vi "GeneralDataRequest.vi"(6 "Enable":bool, 8 "error in (no error)":errorcluster, 10 "Cluster":T2, 11 "VISA Refnum in":refnum<visa-resource-name>) -> (0 "error out":errorcluster, 3 "Sensor data":T1)   [LabVIEW 2020]
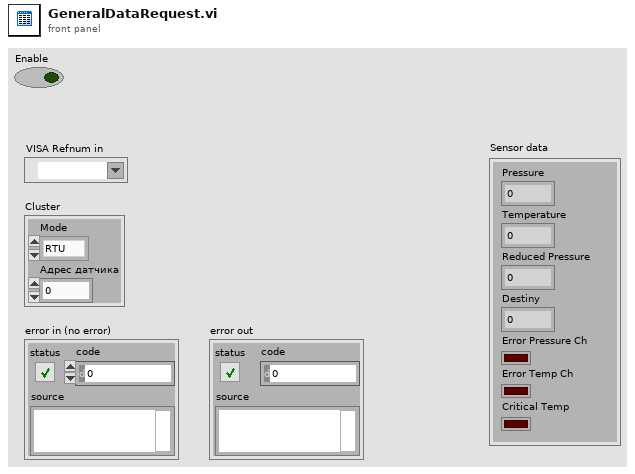
[diagram p1: front panel]
types:
  T1 = cluster{"Pressure":sgl, "Temperature":sgl, "Reduced Pressure":sgl, "Destiny":sgl, "Error Pressure Ch":bool, "Error Temp Ch":bool, "Critical Temp":bool}
  T2 = cluster{"Mode":enum16{"RTU", "ASCII"}, "Адрес датчика":u16}
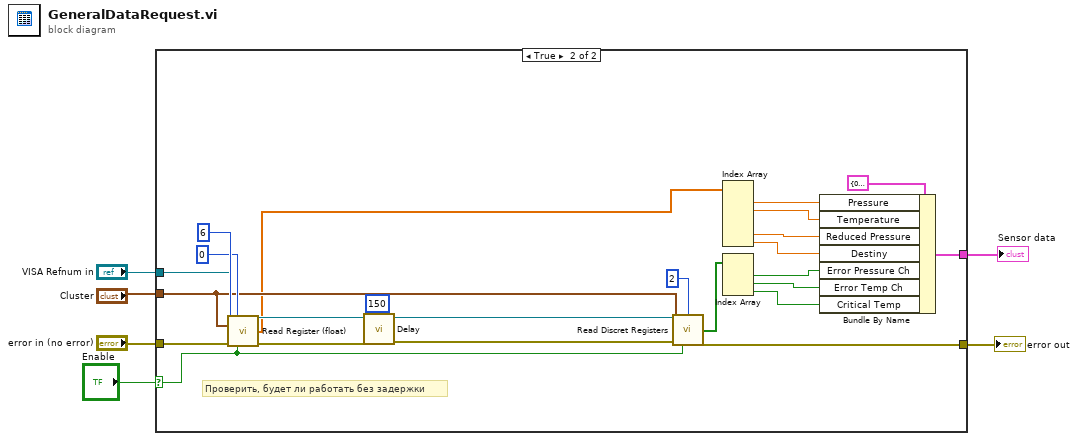
[diagram p0: block diagram]
diagram:
  n1 = case shown="True" "Enable" {
    selector: "Enable" -> [_ w19]
    tunnel: "error in (no error)" -> [w7 w29]
    tunnel: "VISA Refnum in" -> [_ w28]
    tunnel: "Cluster" -> [_ w21]
    tunnel: [w7 w20] -> w3
    tunnel: [_ w12] -> w1
    frame False {
    }
    frame True {
      # "Проверить, будет ли работать без задержки"
      n2 = call "Read Register (float).vi"("Refnum in"=w28, "startReg"=u16 0 ("Holding Register"), "Mode"=w21, "WordCount"=u16 6 ("Holding Register"), "error in (no error)"=w29, "Enable"=w19) -> ("Refnum Out"=w25:refnum<visa-resource-name>, "Data"=w10:sgl[], "error out"=w24:errorcluster)  [unwired: 5 in, 2 out]
      n3 = call "Delay.vi"("milliseconds to wait"=u32 150, "error in (no error)"=w24, "VISA Refnum  In"=w25) -> ("error out"=w23:errorcluster, "VISA Refnum out"=w22:refnum<visa-resource-name>)  [unwired: 7 in]
      n4 = call "Read Discret Registers.vi"("Refnum in"=w22, "Quantity"=u16 2 ("Holding Register"), "Mode"=w21, "error in (no error)"=w23, "Enable"=w19) -> ("Discret Registers"=w16:bool[], "error out"=w20:errorcluster)  [unwired: 7 in, 2 out]
      n5 = Index Array(array=w10) -> (element #1=w18:sgl, element #2=w17:sgl, element #5=w8:sgl, element #6=w9:sgl)  [unwired: 6 in, 2 out]
      n6 = Index Array(array=w16) -> (element #1=w15:bool, element #2=w14:bool, element #3=w13:bool)  [unwired: 3 in]
      n7 = Bundle By Name(cluster=T1 {"Pressure"=0.0, "Temperature"=0.0, "Reduced Pressure"=0.0, "Destiny"=0.0, "Error Pressure Ch"=FALSE, "Error Temp Ch"=FALSE, "Critical Temp"=FALSE} ("Sensor data"), "Pressure"=w18, "Temperature"=w17, "Reduced Pressure"=w8, "Destiny"=w9, "Error Pressure Ch"=w15, "Error Temp Ch"=w14, "Critical Temp"=w13) -> (w12:T1)
    }
  }
  "error out" <- w3
  "Sensor data" <- w1
